vi "Running.vi"(8 "error in (no error)":errorcluster, 11 "CIFCorePlugin in":refnum<class "CIFCorePlugin.lvclass">) -> (0 "error out":errorcluster, 2 "Destroy":bool, 3 "CIFCorePlugin out":refnum<class "CIFCorePlugin.lvclass">)   [LabVIEW 2021, in "CIFCorePlugin.lvclass"]
uses:
  CIFCorePlugin.lvclass
  CIFCorePlugin.lvclass/CIFCorePlugin.ctl
  Typedef/Energized States.ctl
  CIFUtilities/CIFOutOfBand/CIFOutOfBand.lvclass/CIFOutOfBand.ctl
  CIFCoreOOB/OOB_Tx/Send/Update Status Command.vi
  CIFCoreOOB/OOB_Tx/Send/Update Override Command.vi
  CIFUtilities/CIFOutOfBand/Write OOB DVR.vi
  CIFUtilities/CIFOutOfBand/Utilities/Command to Bitwise Command.vi
  CIFUtilities/CIFOutOfBand/Accessors/Read Local OOB Data.vi
  CIFUtilities/CIFOutOfBand/Accessors/Write Local OOB Data.vi
  CIFCoreOOB/OOB_Tx/CIFCoreOOB_Tx.lvclass
  D:/dev/CIF-LVCore/src/CIFUtilities/CIFOutOfBand/CIFOutOfBand.lvclass
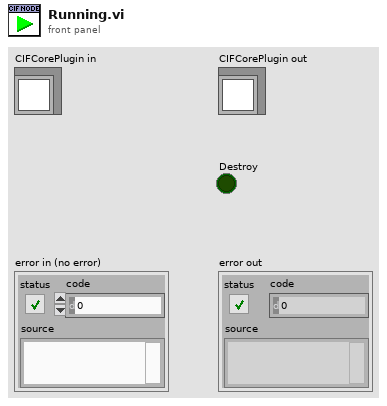
[diagram p1: front panel]
types:
  T1 = typedef "CIFCorePlugin.lvclass/Energized States.ctl" = enum16{"Listen", "Prepare", "Execute", "Housekeep", "Cleanup", "Destroy"}
  T2 = typedef "CIFCorePlugin.lvclass/Running State Logic.ctl" = enum16{"Execute", "Housekeep", "Cleanup", "Error", "Destroy"}
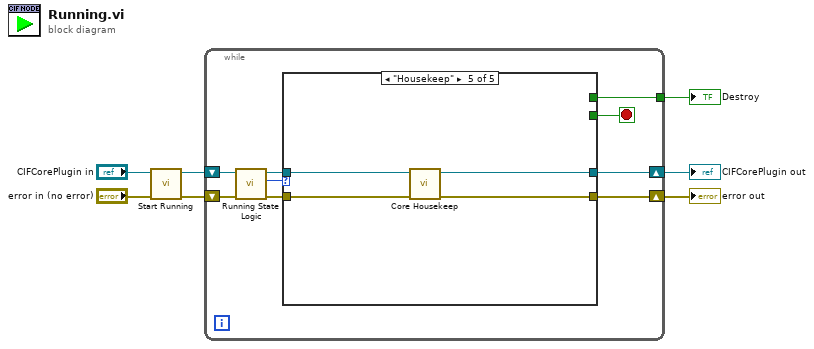
[diagram p0: block diagram]
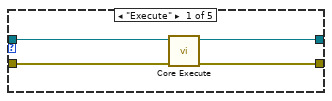
[diagram p2: hidden frame]
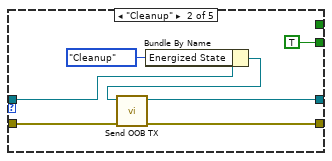
[diagram p3: hidden frame]
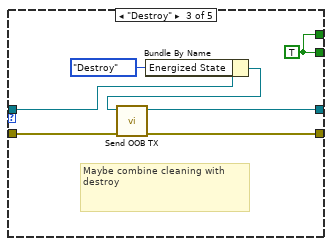
[diagram p4: hidden frame]
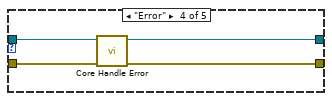
[diagram p5: hidden frame]
diagram:
  n1 = call "Start Running.vi"("error in (no error)"="error in (no error)", "CIFCorePlugin in"="CIFCorePlugin in") -> ("error out"=w1:errorcluster, "CIFCorePlugin out"=w3:refnum<class "CIFCorePlugin.lvclass">)  [unwired: 8 in]
  n2 = while {
    shift-right: [w11] -> w6
    shift-left: w3 -> [w16]
    shift-right: [w10] -> w5
    shift-left: w1 -> [w15]
    tunnel: [w8] -> w7
    stop <- w9 stop-if-true
    n3 = call "Running State Logic.vi"("error in (no error)"=w15, "CIFCorePlugin in"=w16) -> ("error out"=w12:errorcluster, "Running State Logic"=w14:T2, "CIFCorePlugin out"=w13:refnum<class "CIFCorePlugin.lvclass">)  [unwired: 7 in]
    n4 = case shown="\"Housekeep\"" w14 {
      tunnel: w13 -> [w19 w22 w30 w38 w42]
      tunnel: w12 -> [w20 w26 w34 w37 w41]
      tunnel: [w17 w25 w33 w36 w40] -> w11
      tunnel: [w18 w24 w32 w35 w39] -> w10
      tunnel: [_ TRUE w28 _ _] -> w9
      tunnel: [_ _ w28 _ _] -> w8
      frame "Execute" {
        n5 = call "Core Execute.vi"("error in (no error)"=w20, "CIFTemplateNode in"=w19) -> ("error out"=w18:errorcluster, "CIFTemplateNode out"=w17:refnum<class "CIFCorePlugin.lvclass">)  [unwired: 8 in]
      }
      frame "Cleanup" {
        n6 = Bundle By Name(cluster=w22, "Energized State"=Energized_States."Cleanup") -> (w21:refnum<class "CIFCorePlugin.lvclass">)
        n7 = call "Send OOB TX.vi"("error in (no error)"=w26, "CIFCorePlugin in"=w21) -> ("error out"=w24:errorcluster, "CIFCorePlugin out"=w25:refnum<class "CIFCorePlugin.lvclass">)  [unwired: 8 in]
      }
      frame "Destroy" {
        w28 = TRUE
        # "Maybe combine cleaning with destroy"
        n8 = Bundle By Name(cluster=w30, "Energized State"=Energized_States."Destroy") -> (w29:refnum<class "CIFCorePlugin.lvclass">)
        n9 = call "Send OOB TX.vi"("error in (no error)"=w34, "CIFCorePlugin in"=w29) -> ("error out"=w32:errorcluster, "CIFCorePlugin out"=w33:refnum<class "CIFCorePlugin.lvclass">)  [unwired: 8 in]
      }
      frame "Error" {
        n10 = call "Core Handle Error.vi"("error in (no error)"=w37, "CIFTemplateNode in"=w38) -> ("error out"=w35:errorcluster, "CIFTemplateNode out"=w36:refnum<class "CIFCorePlugin.lvclass">)  [unwired: 8 in]
      }
      frame "Housekeep" {
        n11 = call "Core Housekeep.vi"("error in (no error)"=w41, "CIFTemplateNode in"=w42) -> ("error out"=w39:errorcluster, "CIFTemplateNode out"=w40:refnum<class "CIFCorePlugin.lvclass">)  [unwired: 8 in]
      }
    }
  }
  "error out" <- w5
  "CIFCorePlugin out" <- w6
  "Destroy" <- w7
